vi "State Machine.vi"() -> ()   [LabVIEW 2009]
doc: "Ce VI est un modèle de machine à états. Remplacez Processus 1 et Processus 2 par vos états. Pour ajouter d'autres processus, modifiez la constante énumération à définition de type. L'ordre de l'énumération doit correspondre à celui du cluster."
uses:
  State Enum.ctl
panel:
  in  "Menu":T1
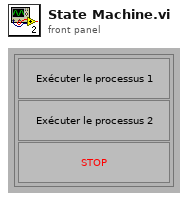
[diagram p1: front panel]
types:
  T1 = cluster{"Processus 1":bool, "Processus 2":bool, "stop":bool}
  T2 = typedef "State Enum.ctl" = enum32{"Inactif", "Processus 1", "Processus 2", "Arrêt"}
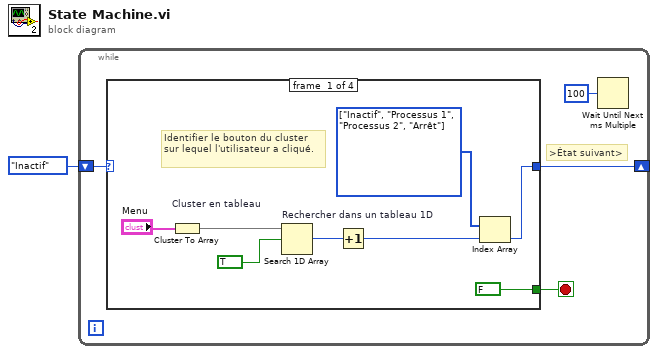
[diagram p0: block diagram]
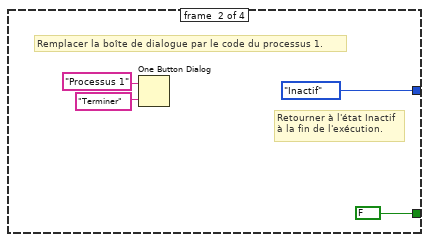
[diagram p2: hidden frame]
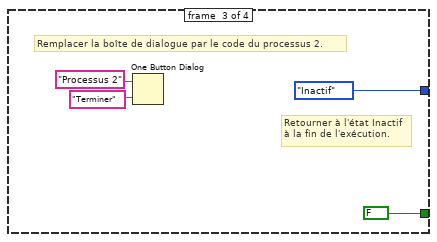
[diagram p3: hidden frame]
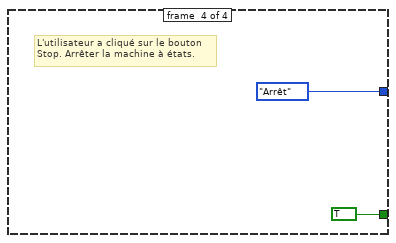
[diagram p4: hidden frame]
diagram:
  n1 = while "Boucle While" {
    shift-right: [w4] -> _
    shift-left: State_Enum."Inactif" ("Enum") -> [w5]
    stop <- w3 stop-if-true
    # ">État suivant>"
    n2 = case "Structure Condition" shown="\"Inactif\", Par défaut" w5 {
      tunnel: [w6 State_Enum."Inactif" ("Enum") State_Enum."Inactif" ("Enum") State_Enum."Arrêt" ("Enum")] -> w4
      tunnel: [FALSE FALSE FALSE TRUE] -> w3
      frame #0 {
        w7 = T2[] [enum."Inactif", enum."Processus 1", enum."Processus 2", enum."Arrêt"] items=["Inactif", "Processus 1", "Processus 2", "Arrêt"]
        # "Identifier le bouton du cluster sur lequel l'utilisateur a cliqué."
        n3 = Cluster To Array "Cluster en tableau"(cluster="Menu") -> (array=w12:bool[])
        n4 = Search 1D Array "Rechercher dans un tableau 1D"(1D array=w12, element=TRUE) -> (index of element=w9:i32)  [unwired: 1 in]
        n5 = Increment(x=w9) -> (x+1=w8:i32)
        n6 = Index Array(array=w7, index=w8) -> (element=w6:T2)
      }
      frame #1 {
        # "Retourner à l'état Inactif\nà la fin de l'exécution."
        # "Remplacer la boîte de dialogue par le code du processus 1."
        n7 = One Button Dialog(message="Processus 1", button name ("OK")="Terminer") -> ()  [unwired: 1 out]
      }
      frame #2 {
        # "Remplacer la boîte de dialogue par le code du processus 2."
        # "Retourner à l'état Inactif\nà la fin de l'exécution."
        n8 = One Button Dialog(message="Processus 2", button name ("OK")="Terminer") -> ()  [unwired: 1 out]
      }
      frame #3 {
        # "L'utilisateur a cliqué sur le bouton\nStop. Arrêter la machine à états."
      }
    }
    n9 = Wait Until Next ms Multiple ("Attendre un multiple de ms")(millisecond multiple=u32 100) -> ()  [unwired: 1 out]
  }
